vi "_095.vi"() -> ()   [LabVIEW 2020]
panel:
  out "Numeric":i32
  # "What value will be displayed in the Numeric indicaator on the front panel after this code executes?"
  # "Workflow:"
  # "In 1st frame 5 will write in local variable & then in 2nd frame The readed value was written and connected to increment function and it will incremented +1 , finally in last frame value was 6"
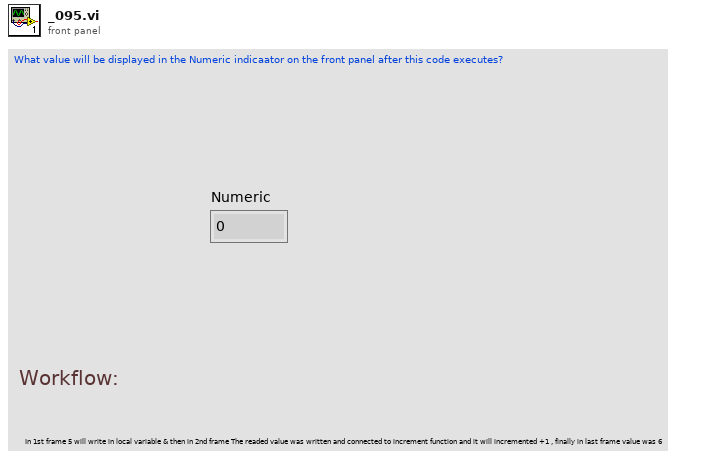
[diagram p1: front panel]
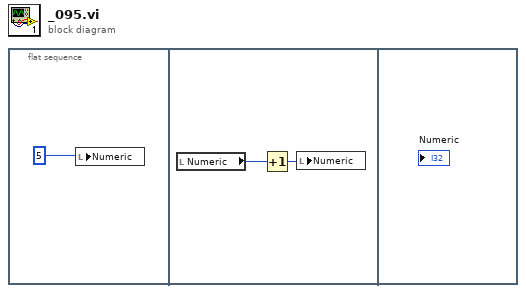
[diagram p0: block diagram]
diagram:
  n1 = flat-sequence {
    frame #0 {
      n2 = local write "Numeric"(5) -> ()
    }
    frame #1 {
      n3 = local read "Numeric"() -> (w3:i32)
      n4 = Increment(x=w3) -> (x+1=w2:i32)
      n5 = local write "Numeric"(w2) -> ()
    }
    frame #2 {
    }
  }
